vi "service status.vi"(8 "error in":errorcluster, 11 "Service Name":string="MSSQL$SQLEXPRESS") -> (0 "error out":errorcluster, 1 "Array":string[](array[string]), 2 "Status Number":i32, 3 "Status":i32(ring)=1 items=["Stopped"=1, "StartPending"=2, "StopPending"=3, "Running"=4, "ContinuePending"=5, "PausePending"=6, "Paused"=7])   [LabVIEW 2017]
doc: "This VI is used to find Status of Windows Services for SQL is start, wait for 180 seconds and if in this time it not found running then application sends not running status to main program."
uses:
  System.ServiceProcess
  ac4aeb18-7f19-4ac4-a43e-f82d8e4d68fc.vi
panel:
  out "Loading":i32(slide)=1 scale=0.0..300.0
  out "Service Number":i32
  out "element":string="MSSQL$SQLEXPRESS"
  in  "reference":refnum<k24>
  # "Loading.............."
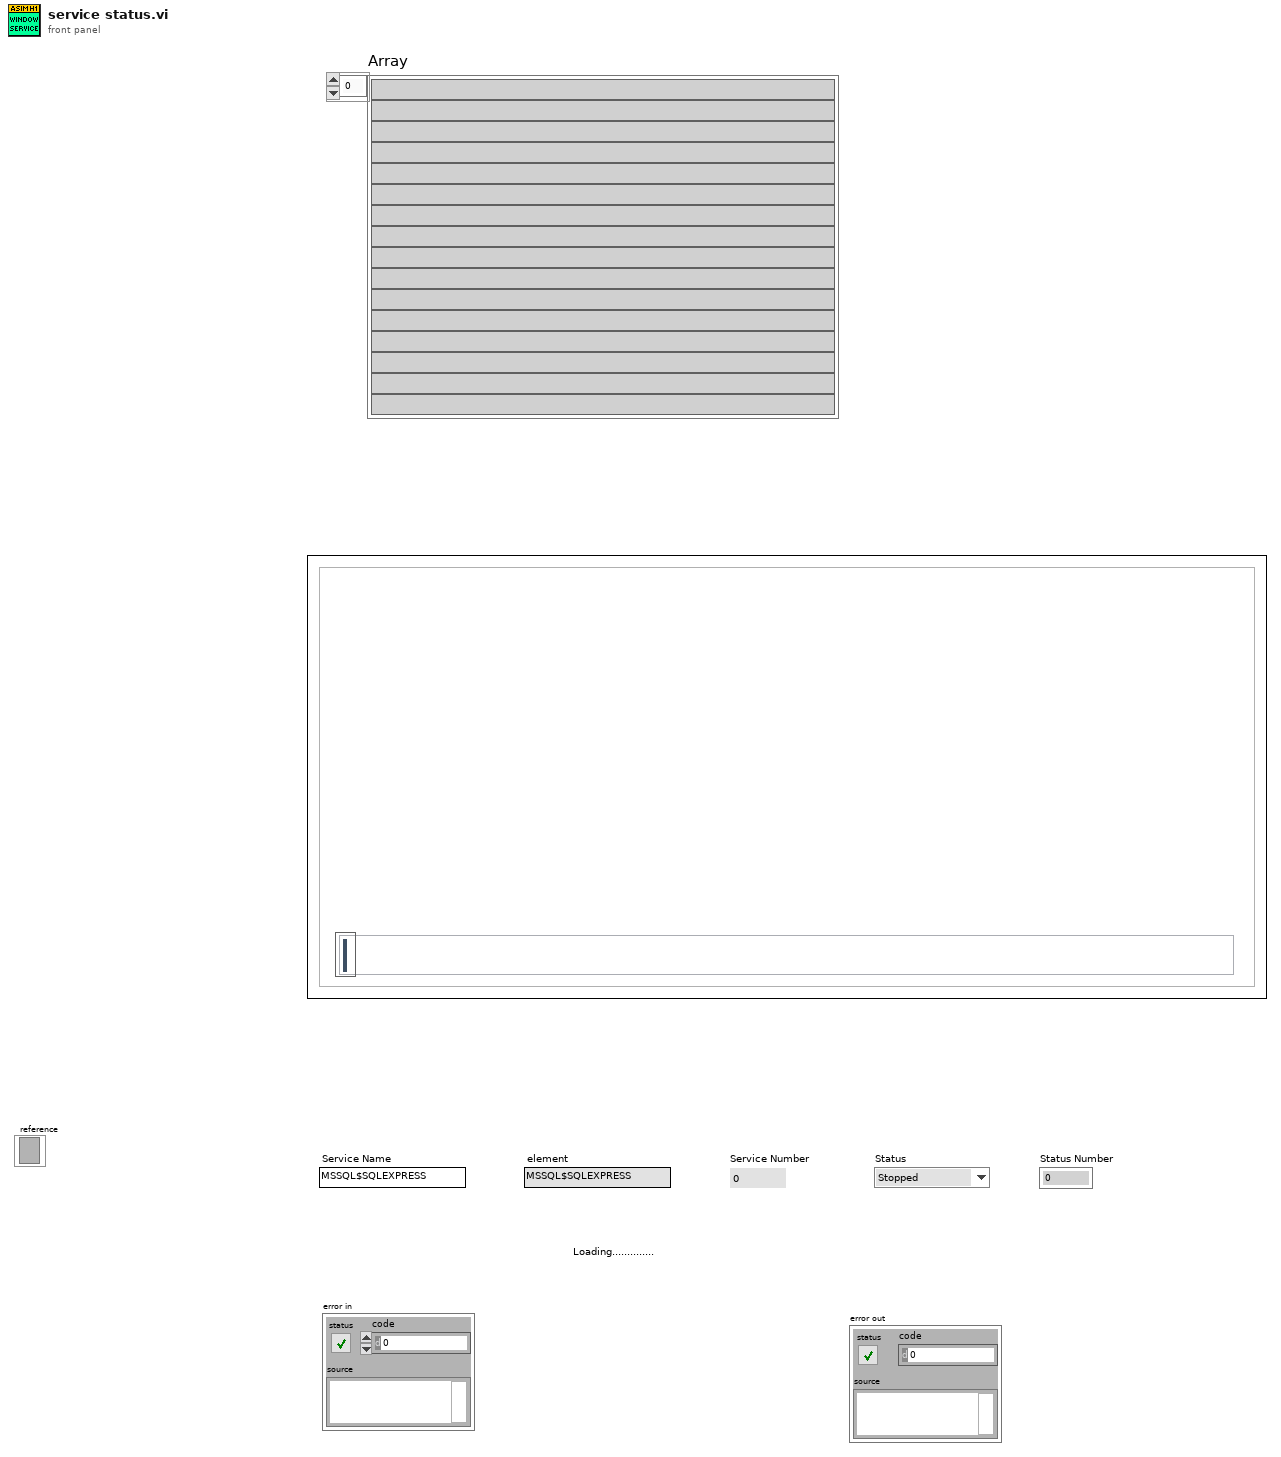
[diagram p1: front panel]
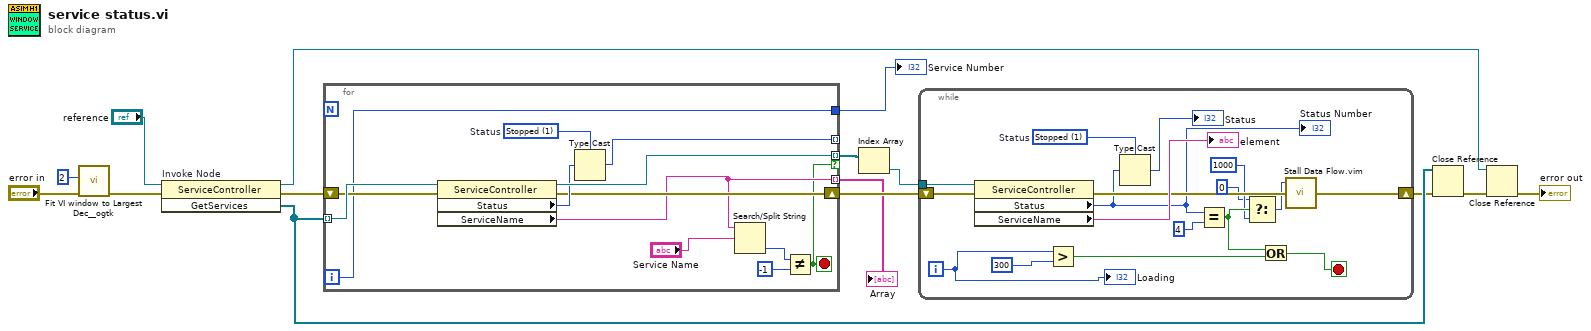
[diagram p0: block diagram]
diagram:
  n1 = call "Fit VI window to Largest Dec__ogtk.vi"("error in (no error)"="error in", "border spacing (2 px)"=2) -> ("error out"=w5:errorcluster)  [unwired: 4 in, 1 out]
  n2 = invoke on="Invoke Node" class="ServiceController" method="GetServices"(reference="reference", error in=w5) -> (reference out=w8:refnum<k24>, error out=w14:errorcluster, "GetServices"=w11:refnum<k24>[])  [unwired: 1 in]
  n3 = for {
    tunnel: w11 -> [w28] mode=indexing
    tunnel: [w27] -> w3 mode=indexing if=w16
    tunnel: [w21] -> w1 mode=indexing
    tunnel: [w24] -> _ mode=indexing
    shift-right: [w22] -> w10
    shift-left: w14 -> [w23]
    tunnel: [w17] -> w7
    i -> [w17]
    stop <- w16 stop-if-true
    w26 = 1 items=["Stopped"=1, "StartPending"=2, "StopPending"=3, "Running"=4, "ContinuePending"=5, "PausePending"=6, "Paused"=7]  # Status
    n4 = property class="ServiceController"(reference=w28, error in=w23) -> (reference out=w27:refnum<k24>, error out=w22:errorcluster, "Status"=w25:i32, "ServiceName"=w21:string)
    n5 = Type Cast(type=w26, x=w25) -> (*(type *) &x=w24:i32)
    n6 = Search/Split String(string=w21, search string/char (-)="Service Name") -> (offset of match=w18:i32)  [unwired: 1 in, 2 out]
    n7 = Not Equal?(x=w18, y=-1) -> (x != y?=w16:bool)
  }
  "Service Number" <- w7
  "Array" <- w1
  n8 = Index Array(array=w3) -> (element=w2:refnum<k24>)  [unwired: 1 in]
  n9 = while {
    tunnel: w2 -> [w45]
    shift-right: [w39] -> w9
    shift-left: w10 -> [w44]
    i -> [w29]
    stop <- w38 stop-if-true
    w42 = 1 items=["Stopped"=1, "StartPending"=2, "StopPending"=3, "Running"=4, "ContinuePending"=5, "PausePending"=6, "Paused"=7]  # Status
    n10 = property class="ServiceController"(reference=w45, error in=w44) -> (error out=w40:errorcluster, "Status"=w30:i32, "ServiceName"=→"element":string)  [unwired: 1 out]
    "Status Number" <- w30
    n11 = Greater?(x=w29, y=300) -> (0:w36:bool)
    n12 = Type Cast(type=w42, x=w30) -> (*(type *) &x=→"Status":i32)
    n13 = Equal?(x=w30, y=4) -> (x = y?=w33:bool)
    n14 = Select(t=u32 0, s=w33, f=u32 1000 ("milliseconds to wait")) -> (s? t:f=w34:u32)
    n15 = Or(x=w33, y=w36) -> (x .or. y?=w38:bool)
    n16 = call "Stall Data Flow.vim"("value in"=w40, "milliseconds to wait"=w34) -> ("value out"=w39:errorcluster)  [unwired: 1 out]
    "Loading" <- w29
  }
  n17 = Close Reference(reference=w11, error in (no error)=w9) -> (error out=w13:errorcluster)
  n18 = Close Reference(reference=w8, error in (no error)=w13) -> (error out=→"error out":errorcluster)
